vi "Get Zenoh Path.vi"() -> (4 "Library Path":path)   [LabVIEW 2021, in "Zenoh.lvclass"]
uses:
  Zenoh.lvclass
  Zenoh.lvclass/Zenoh.ctl
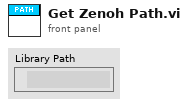
[diagram p1: front panel]
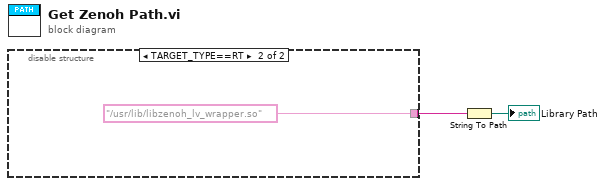
[diagram p0: block diagram]
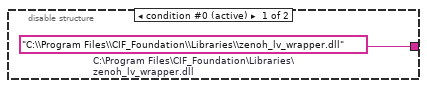
[diagram p2: hidden frame]
diagram:
  n1 = disable-structure shown="TARGET_TYPE==RT" {
    disable-tunnel: [w3 "/usr/lib/libzenoh_lv_wrapper.so"] -> w2
    frame condition #0 (active) {
      w3 = "C:\\Program Files\\CIF_Foundation\\Libraries\\zenoh_lv_wrapper.dll"  # C:\Program Files\CIF_Foundation\Libraries\zenoh_lv_wrapper.dll
    }
    frame condition #1 {
    }
  }
  n2 = String To Path(string=w2) -> (path=→"Library Path":path)
